vi "get_selfTestResult.vi"(0 "HGF_Device_SelfTest":refnum<class "HGF_Device_SelfTest.lvclass">, 5 "error in (no error)":errorcluster) -> (14 "dup HGF_Device_SelfTest":refnum<class "HGF_Device_SelfTest.lvclass">, 16 "passed?":bool, 17 "resultCode":i32, 18 "resultMessage":string, 19 "error out":errorcluster)   [LabVIEW 2014, in "HGF_DeviceBaseClasses.lvlib" / "HGF_Device_SelfTest.lvclass"]
doc: "This VI returns the SelfTest result data."
uses:
  HGF_Device_SelfTest.lvclass
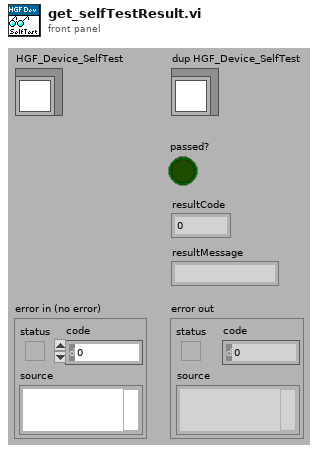
[diagram p1: front panel]
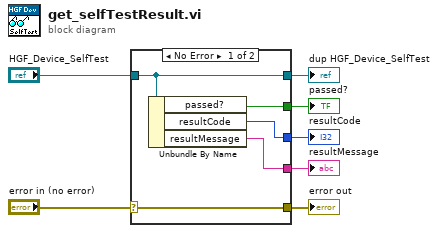
[diagram p0: block diagram]
diagram:
  n1 = case shown="No Error" "error in (no error)" {
    selector: "error in (no error)" -> [w12 w13]
    tunnel: [w12 w13] -> w6
    tunnel: [w11 w14] -> w4
    tunnel: "HGF_Device_SelfTest" -> [w11 w14]
    tunnel: [w10 _] -> w3
    tunnel: [w9 _] -> w2
    tunnel: [w8 _] -> w1
    frame No Error {
      n2 = Unbundle By Name(w11) -> ("passed?"=w10:bool, "resultCode"=w9:i32, "resultMessage"=w8:string)
    }
    frame Error {
    }
  }
  "error out" <- w6
  "dup HGF_Device_SelfTest" <- w4
  "passed?" <- w3
  "resultCode" <- w2
  "resultMessage" <- w1
